vi "wyjscia joya.vi"(8 "szukaj joy":bool, 9 "index joya jazda":i32=2) -> (0 "error out":errorcluster, 1 "wyjscia joya":T3, 2 "axis info":T4, 3 "number":u32, 4 "Refnum out":refnum<k1>)   [LabVIEW 2015]
uses:
  Wyjscia joya.ctl
  <vilib>/Utility/inputDevices.llb/joystickAcquire.vi
  <vilib>/MakerHub/Xbox-One-Controller/LMH-Xbox-One-Controller.lvlib
panel:
  out "direction info":T1
  out "button info":T2
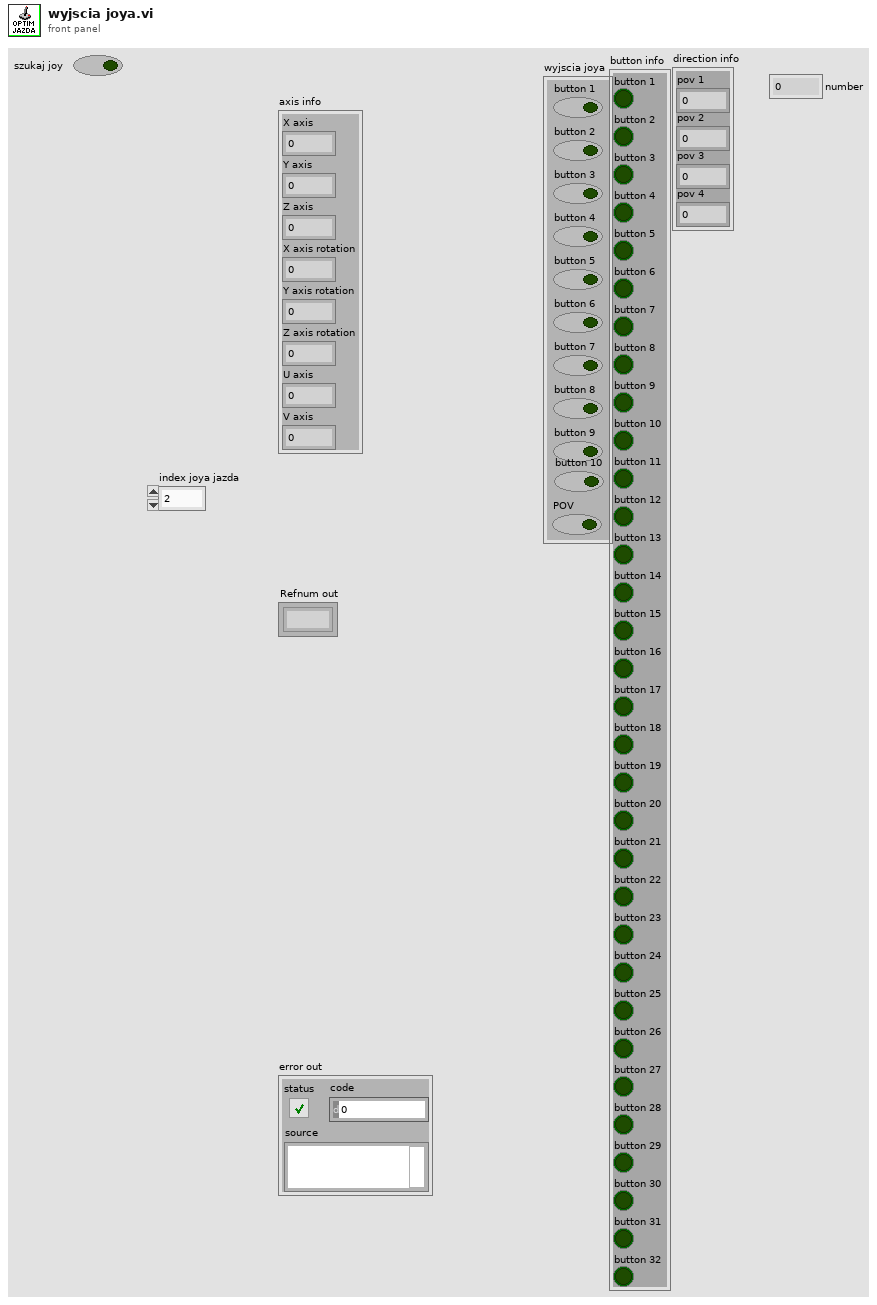
[diagram p1: front panel]
types:
  T1 = cluster{"pov 1":i32, "pov 2":i32, "pov 3":i32, "pov 4":i32}
  T2 = cluster{"button 1":bool, "button 2":bool, "button 3":bool, "button 4":bool, "button 5":bool, "button 6":bool, "button 7":bool, "button 8":bool, "button 9":bool, "button 10":bool, "button 11":bool, "button 12":bool, "button 13":bool, "button 14":bool, "button 15":bool, "button 16":bool, "button 17":bool, "button 18":bool, "button 19":bool, "button 20":bool, "button 21":bool, "button 22":bool, "button 23":bool, "button 24":bool, "button 25":bool, "button 26":bool, "button 27":bool, "button 28":bool, "button 29":bool, "button 30":bool, "button 31":bool, "button 32":bool}
  T3 = typedef "Wyjscia joya.ctl" = cluster{"button 1":bool, "button 2":bool, "button 3":bool, "button 4":bool, "button 5":bool, "button 6":bool, "button 7":bool, "button 8":bool, "button 9":bool, "POV":bool, "button 10":bool}
  T4 = cluster{"X axis":i32, "Y axis":i32, "Z axis":i32, "X axis rotation":i32, "Y axis rotation":i32, "Z axis rotation":i32, "U axis":i32, "V axis":i32}
  T5 = typedef "LMH-Xbox-One-Controller.lvlib/Xbox Controller Device.ctl" = cluster{"Device Index":i32, "Device Name":string}
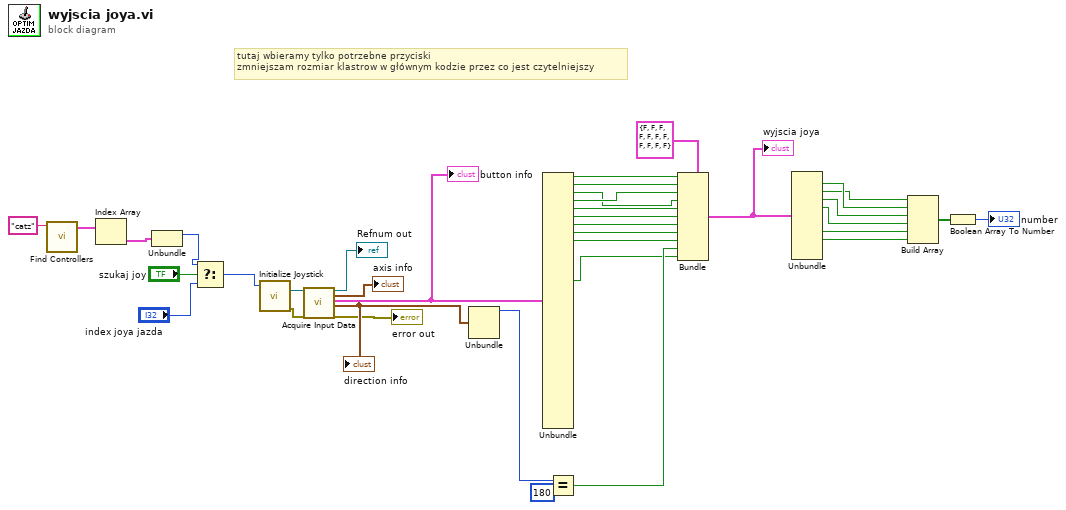
[diagram p0: block diagram]
diagram:
  # "tutaj wbieramy tylko potrzebne przyciski \nzmniejszam rozmiar klastrow w głównym kodzie przez co jest czytelniejszy"
  n1 = call <vilib>:"Find Controllers.vi"("search string/char (-)"="catz") -> ("Xbox Controllers"=w4:T5[])  [unwired: 9 in, 1 out]
  n2 = Index Array(array=w4) -> (element=w3:T5)  [unwired: 1 in]
  n3 = Unbundle(w3) -> ("Device Index"=w2:i32)  [unwired: 1 out]
  n4 = Select(t=w2, s="szukaj joy", f="index joya jazda") -> (s? t:f=w6:i32)
  n5 = call <vilib>:"Initialize Joystick.vi"("device index"=w6) -> ("error out"=w22:errorcluster, "device ID"=w23:refnum<k1>)  [unwired: 9 in]
  n6 = call-poly <vilib>:"Acquire Input Data.vi"("device ID"=w23, "error in (no error)"=w22) -> ("device ID"=→"Refnum out":refnum<k1>, "axis info"=→"axis info":T4, "button info"=w35:T2, "direction info"=w37:T1, "error out"=→"error out":errorcluster)  [unwired: 13 in]
  "button info" <- w35
  "direction info" <- w37
  n7 = Unbundle(w37) -> ("pov 1"=w19:i32)  [unwired: 3 out]
  n8 = Unbundle(w35) -> ("button 1"=w21:bool, "button 2"=w31:bool, "button 3"=w17:bool, "button 4"=w18:bool, "button 5"=w30:bool, "button 6"=w29:bool, "button 7"=w28:bool, "button 8"=w27:bool, "button 9"=w26:bool, "button 14"=w20:bool)  [unwired: 22 out]
  n9 = Equal?(x=w19, y=180) -> (x = y?=w25:bool)
  n10 = Bundle(cluster=T3 {"button 1"=FALSE, "button 2"=FALSE, "button 3"=FALSE, "button 4"=FALSE, "button 5"=FALSE, "button 6"=FALSE, "button 7"=FALSE, "button 8"=FALSE, "button 9"=FALSE, "POV"=FALSE, "button 10"=FALSE}, "button 1"=w21, "button 2"=w31, "button 3"=w18, "button 4"=w17, "button 5"=w30, "button 6"=w29, "button 7"=w28, "button 8"=w27, "button 9"=w26, "POV"=w25, "button 10"=w20) -> (w10:T3)
  "wyjscia joya" <- w10
  n11 = Unbundle(w10) -> ("button 2"=w15:bool, "button 3"=w14:bool, "button 4"=w13:bool, "button 5"=w12:bool, "button 8"=w11:bool, "button 9"=w8:bool)  [unwired: 5 out]
  n12 = Build Array(w14, w15, w13, w12, w11, w8) -> (w16:bool[])
  n13 = Boolean Array To Number(Boolean array=w16) -> (number=→"number":u32)
